vi "Sensor_Reference_Sensor_v1.1.vi"() -> ()   [LabVIEW 2012]
doc: "This example VI demonstrates setting up a scan list and taking a reading using the advanced VIs. For more information about the different types of VIs, see the descriptions below.\n\nEven though only two types of measurements are shown, all six types can be configured in the same way. Likewise, this VI does not show every available configurable option for voltage and resistance.\n\n====================\nSetting up and performing a scan\n====================\nThe HP34970A provides commands for setting up a scan in three ways that differ in their complexity and the amount of control offered:\n\n1. Advanced:\nEvery aspect of the measurement, scan, scan list, and read is put in a different command to allow the greatest flexibility. For example, using the advanced configure VIs, you can set up a scan list consisting of different measurement types on different channels. The \"HP34970A Advanced Scan Example.vi\" demonstrates usage of these VIs.\n\n2. Medium:\nThe instrument also offers a command that wraps up configuring individual channels and the scan list. This is represented in the driver by \"HP34970A Conf EZ.vi\". This driver specifically replaces use of the advanced configure measurement VIs and configure scan list VIs. For more information, refer to the context help for the Conf EZ VI.\n\n3. Easiest:\nThe entire configuration, scan, and read are wrapped up into one command to the instrument. This is provided in this driver as the \"EZ\" VIs, which are in the Data subpalette of the HP34970A's driver palette. The \"HP34970A EZ Scan Example.vi\" demonstrates the EZ VI's usage."
uses:
  <instrlib>/Agilent 34970/Agilent 34970.lvlib
  <vilib>/Analysis/NI_AALPro.lvlib
panel:
  in  "enable autozero":bool=TRUE
  out "real sampling time / ms":dbl[](array[numeric])
  out "size(s)":i32[](array[numeric])
  in  "Sample time set point / s":dbl=0.01
  out "max value":dbl
  out "Waveform Graph 2":T1(graph)
  out "read buffer":string
  in  "Scan Fields":T2={"Include Alarm Data F:(No)"=FALSE, "Include Channel # (F:No)"=FALSE, "Include Time (F:No)"=TRUE, "Include Units (F:No)"=FALSE}
  in  "number of readings":i32=3
  in  "Advanced Config":T3={"Aperture Value (.4)"=0.4, "Aperture (1:Minimum)"=1, "NPLC (1)"=2, "Bandwidth (3 Hz)"=0, "Input Impedance (F:Fixed)"=FALSE, "Integration Time (F:Aperture)"=TRUE} {"Aperture (1:Minimum)" items=["Manual", "Minimum", "Maximum"]; "NPLC (1)" items=[".02", ".2", "1", "2", "10", "20", "100", "200", "Minimum", "Maximum"]; "Bandwidth (3 Hz)" items=["3 Hz", "20 Hz", "200 Hz", "Minimum", "Maximum"]}
  out "measuring time / ms":u32
  out "measurement running":bool
  in  "current transfer ratio":dbl[unit]=1.0 caption="s"
  in  "Reading interval":u32=100
  in  "cancel measurement":bool
  out "standard deviation / %":dbl=nan format="%#_3g"
  out "mean / V":dbl format="%0.5f"
  out "standard deviation / V":dbl format="%0.5f"
  out "Waveform Graph":T1(graph)
  out "Readings":string[][](array[string])
  in  "Range (Volt.)":T4(ring)=enum."10 V"
  in  "Channel List (Volt.)":string="101"
  in  "VISA resource name":refnum<visa-resource-name>="USB0::0x0957::0x2007::MY49004365::INSTR"
  # "Voltage"
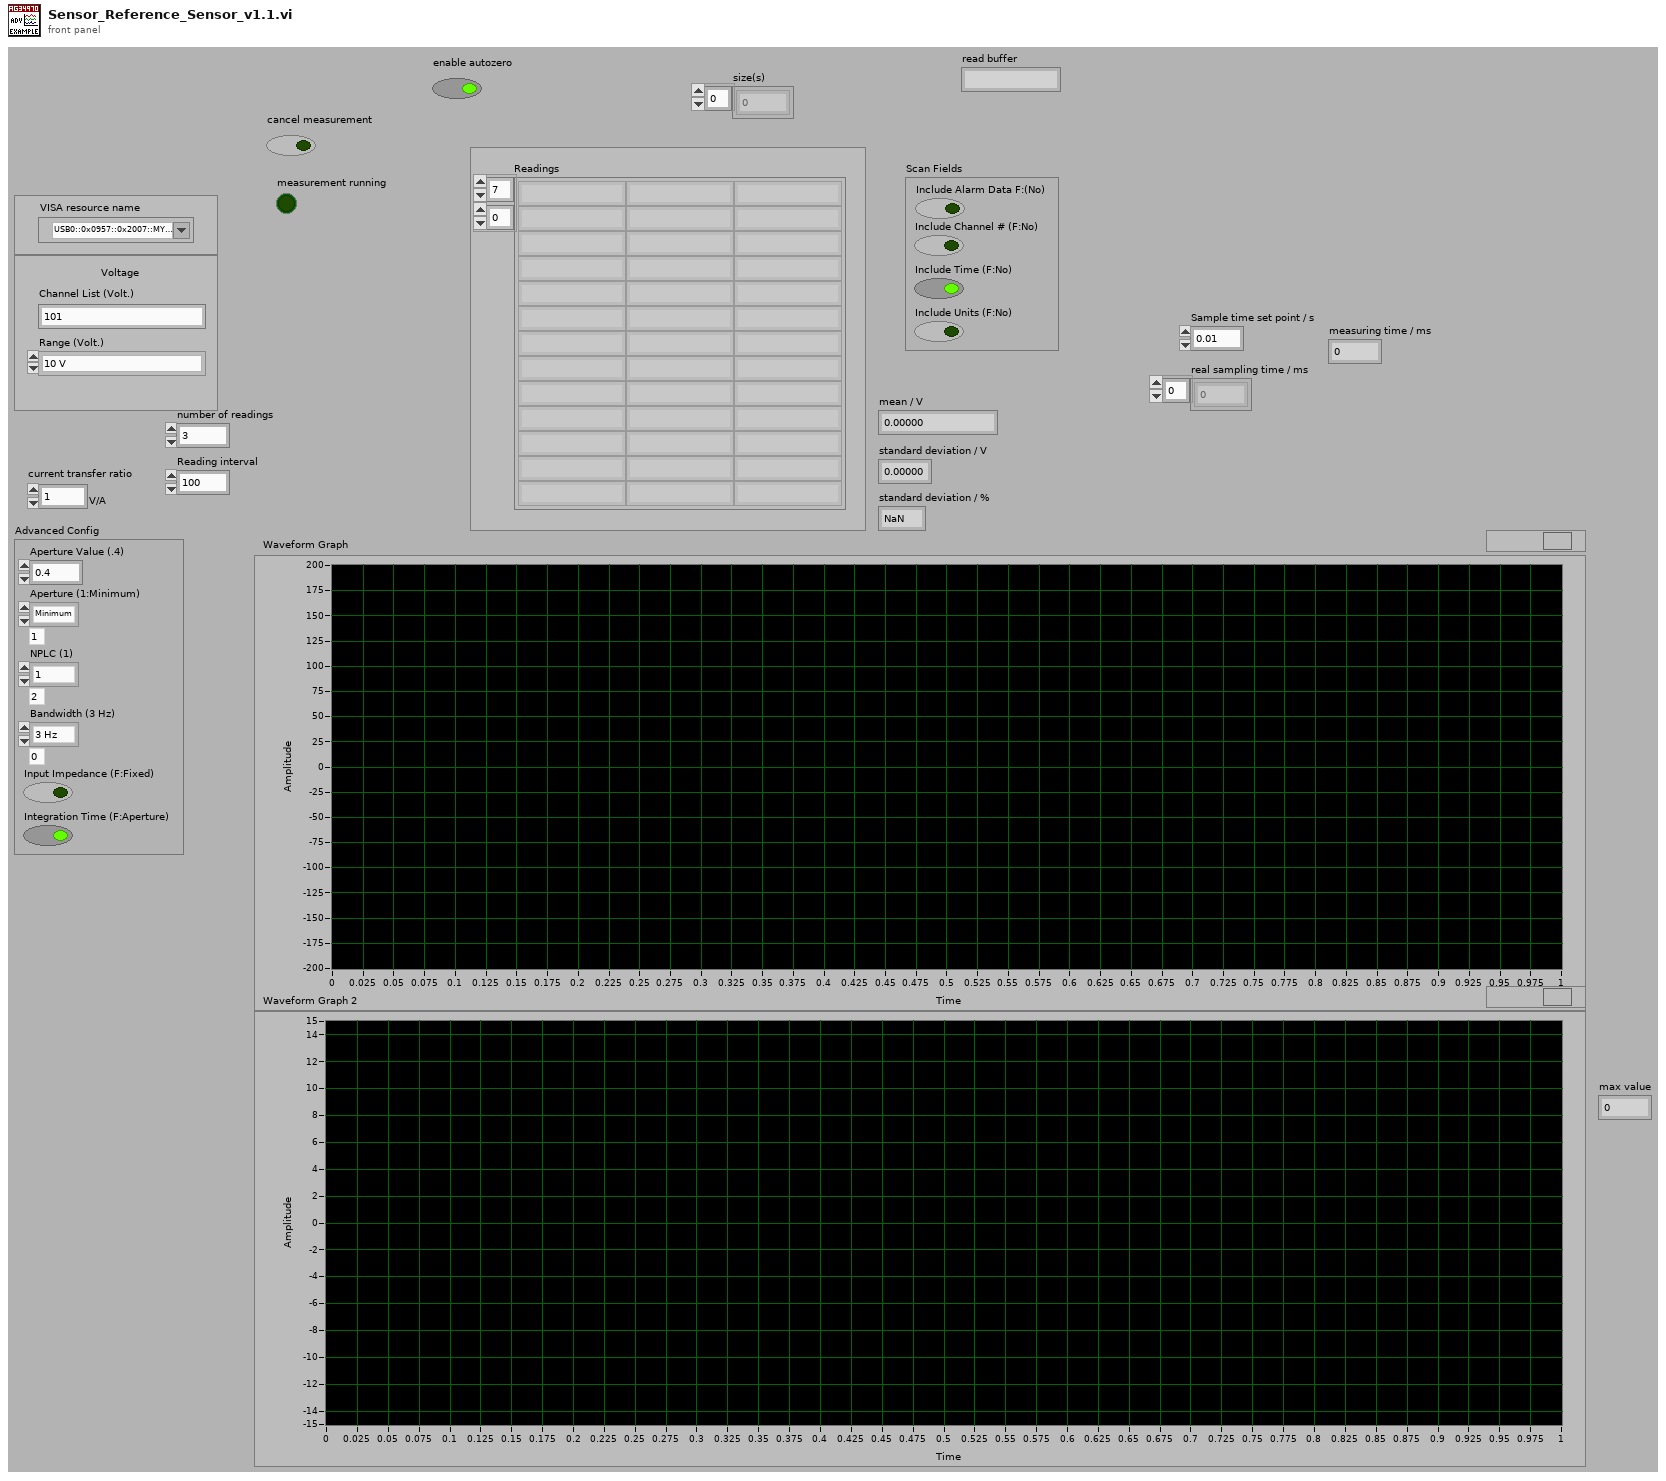
[diagram p1: front panel]
types:
  T1 = cluster{"Interval Value (0)":dbl, "Interval Value (0)":dbl, dbl[]}
  T2 = cluster{"Include Alarm Data F:(No)":bool, "Include Channel # (F:No)":bool, "Include Time (F:No)":bool, "Include Units (F:No)":bool}
  T3 = cluster{"Aperture Value (.4)":dbl, "Aperture (1:Minimum)":u16, "NPLC (1)":u16, "Bandwidth (3 Hz)":u16, "Input Impedance (F:Fixed)":bool, "Integration Time (F:Aperture)":bool}
  T4 = enum16{"100 mV", "1 V", "10 V", "100 V", "300 V", "Minimum", "Maximum"}
  T5 = enum16{"Manual", "Minimum", "Maximum", "Infinity"}
  T6 = enum16{"Remote Trigger", "Immediate Trigger", "Wait for Trigger", "Abort Scan"}
  T7 = enum16{"Bus", "Immediate", "External", "Alarm 1", "Alarm 2", "Alarm 3", "Alarm 4", "Timer"}
  T8 = cluster{"Timeout Value (10000)":u32, "Baud Rate (57600)":enum16{"1200", "2400", "4800", "9600", "19200", "38400", "57600", "115200"}, "Flow Control (1:XON/XOFF)":enum16{"None", "XON / XOFF", "RTS / CTS", "DTR / DSR"}}
  T9 = cluster{dbl, "Sample time set point / s":dbl, dbl[]}
  T10 = cluster{dbl, "Sample time set point / s":dbl, "dX/dt":dbl[]}
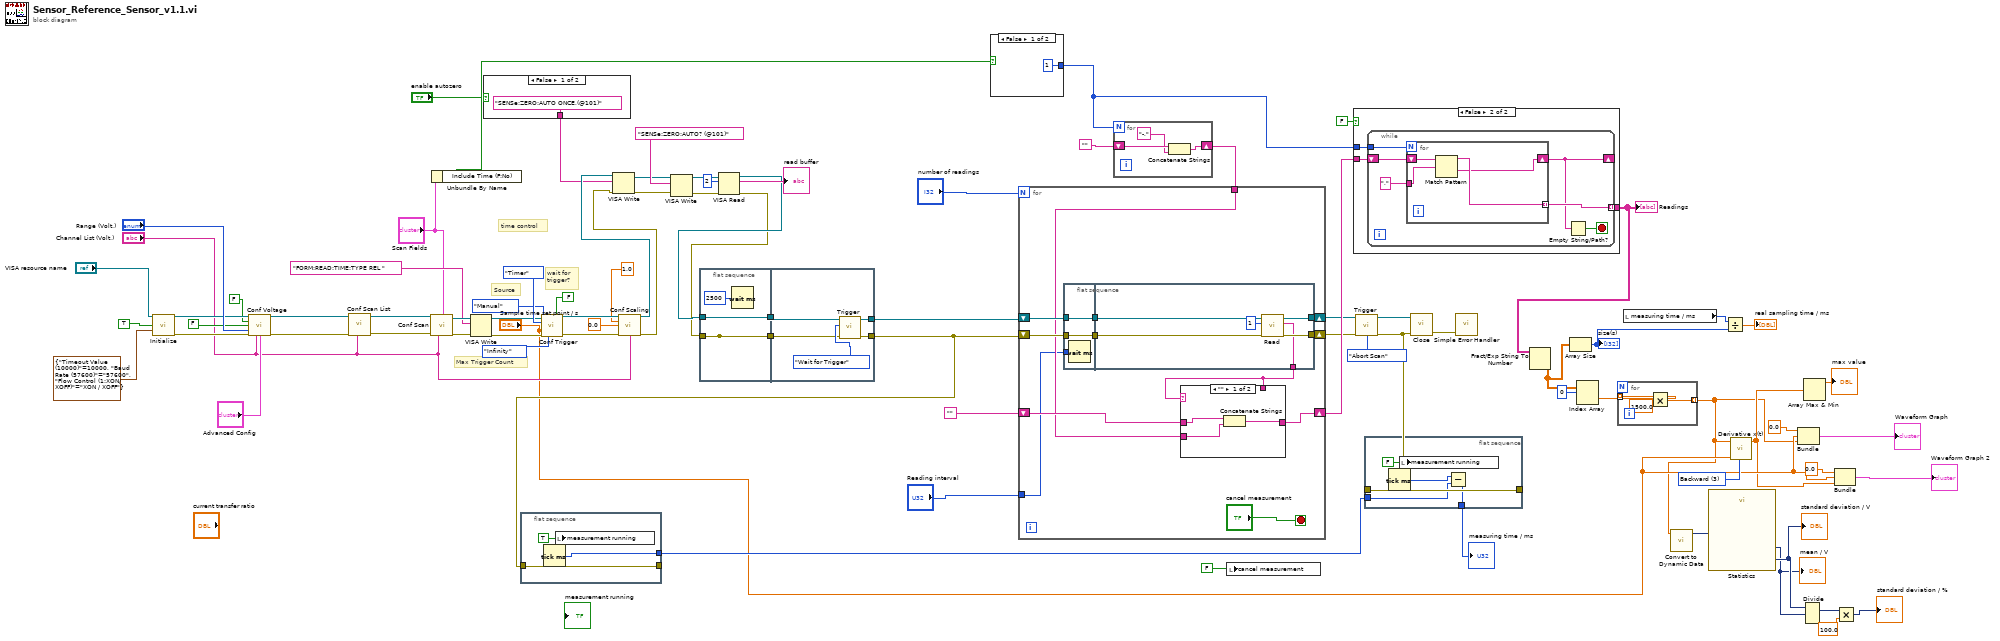
[diagram p0: block diagram]
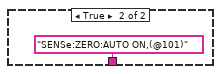
[diagram p2: hidden frame]
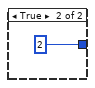
[diagram p3: hidden frame]
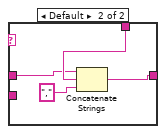
[diagram p4: hidden frame]
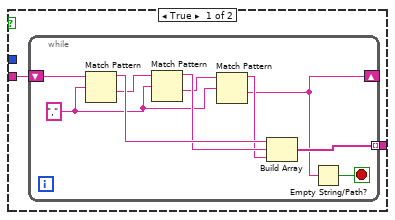
[diagram p5: hidden frame]
diagram:
  w11 = u16 3 items=["2nd Order Central", "4th Order Central", "Forward", "Backward"] ("method")
  # "Max Trigger Count"
  # "wait for \ntrigger?"
  # "time control"
  # "Source"
  n1 = call <instrlib>:"Initialize.vi"("VISA Resource Name"="VISA resource name", "Reset (T: Reset)"=TRUE, "Serial Port Configuration"=T8 {"Timeout Value (10000)"=10000, "Baud Rate (57600)"=enum."57600", "Flow Control (1:XON/XOFF)"=enum."XON / XOFF"}) -> ("VISA Resource Name Out"=w82:refnum<visa-resource-name>, "error out"=w69:errorcluster)  [unwired: 11 in]
  n2 = call <instrlib>:"Conf Voltage.vi"("VISA Resource Name"=w82, "AC/DC (F:DC)"=FALSE, "Autorange? (F:Off)"=FALSE, "Range (6:Max)"="Range (Volt.)", "error in (no error)"=w69, "Channel List (empty)"="Channel List (Volt.)", "Advanced Config"="Advanced Config") -> ("VISA Resource Name Out"=w71:refnum<visa-resource-name>, "error out"=w65:errorcluster)  [unwired: 6 in, 1 out]
  n3 = call <instrlib>:"Conf Scan List.vi"("Scan List (empty)"="Channel List (Volt.)", "error in (no error)"=w65, "VISA Resource Name"=w71) -> ("error out"=w64:errorcluster, "VISA Resource Name Out"=w67:refnum<visa-resource-name>)  [unwired: 6 in, 1 out]
  n4 = call <instrlib>:"Conf Scan.vi"("VISA Resource Name"=w67, "error in (no error)"=w64, "Channel List (empty)"="Channel List (Volt.)", "Scan Fields"="Scan Fields") -> ("VISA Resource Name Out"=w55:refnum<visa-resource-name>, "error out"=w54:errorcluster)  [unwired: 9 in, 1 out]
  n5 = Unbundle By Name("Scan Fields") -> ("Include Time (F:No)"=w37:bool)
  n6 = VISA Write(VISA resource name=w55, write buffer="FORM:READ:TIME:TYPE REL ", error in (no error)=w54) -> (VISA resource name out=w52:refnum<visa-resource-name>, error out=w53:errorcluster)  [unwired: 1 out]
  n7 = case shown="False" "enable autozero" {
    tunnel: ["SENSe:ZERO:AUTO ONCE,(@101)" ("write buffer") "SENSe:ZERO:AUTO ON,(@101)" ("write buffer")] -> w18
    frame False {
    }
    frame True {
    }
  }
  n8 = flat-sequence {
    tunnel: w35 -> [w89]
    tunnel: [w89] -> _
    tunnel: [w88] -> w57
    frame #0 {
      n9 = Tick Count (ms)() -> (millisecond timer value=w88:u32)
      n10 = local write "measurement running"(TRUE ("measurement running")) -> ()
    }
  }
  n11 = call <instrlib>:"Conf Trigger.vi"("VISA Resource Name"=w52, "Wait for Trigger? (F:No)"=FALSE, "Source (1:Immediate)"=T7."Timer", "Time-Scan Interval (1:Min)"=enum16{"Manual", "Minimum", "Maximum"}."Manual", "Interval Value (0)"="Sample time set point / s", "error in (no error)"=w53, "Max Trigger Count (3:Inf)"=T5."Infinity") -> ("VISA Resource Name Out"=w32:refnum<visa-resource-name>, "error out"=w31:errorcluster)  [unwired: 6 in, 1 out]
  n12 = call <instrlib>:"Conf Scaling.vi"("VISA Resource Name"=w32, "Gain (1)"=1.0, "Offset (0)"=0.0, "error in (no error)"=w31, "Channel List (empty)"="Channel List (Volt.)") -> ("VISA Resource Name Out"=w20:refnum<visa-resource-name>, "error out"=w19:errorcluster)  [unwired: 8 in, 1 out]
  n13 = VISA Write(VISA resource name=w20, write buffer=w18, error in (no error)=w19) -> (VISA resource name out=w22:refnum<visa-resource-name>, error out=w21:errorcluster)  [unwired: 1 out]
  n14 = VISA Write(VISA resource name=w22, write buffer="SENSe:ZERO:AUTO? (@101)", error in (no error)=w21) -> (VISA resource name out=w25:refnum<visa-resource-name>, error out=w24:errorcluster)  [unwired: 1 out]
  n15 = flat-sequence {
    tunnel: [w92] -> w17
    tunnel: w16 -> [w92]
    tunnel: [w91] -> _
    tunnel: [w91] -> w15
    tunnel: w14 -> [w91]
    tunnel: [w98] -> w36
    tunnel: [w97] -> w35
    tunnel: w17 -> [w95]
    tunnel: w15 -> [w94]
    frame #0 {
      n16 = Wait (ms)(milliseconds to wait=u32 2500) -> ()  [unwired: 1 out]
    }
    frame #1 {
      n17 = call <instrlib>:"Trigger.vi"("error in (no error)"=w94, "Command (0:Rem Trig)"=T6."Wait for Trigger", "VISA Resource Name"=w95) -> ("error out"=w97:errorcluster, "VISA Resource Name Out"=w98:refnum<visa-resource-name>)  [unwired: 7 in]
    }
  }
  n18 = VISA Read(VISA resource name=w25, byte count=u32 2, error in (no error)=w24) -> (VISA resource name out=w16:refnum<visa-resource-name>, read buffer=→"read buffer":string, error out=w14:errorcluster)  [unwired: 1 out]
  n19 = case shown="False" w37 {
    tunnel: [1 2] -> w41
    frame False {
    }
    frame True {
    }
  }
  n20 = for {
    N: w41 -> [_]
    shift-right: [w101] -> w39
    shift-left: "" -> [w103]
    n21 = Concatenate Strings(w103, "-," ("string")) -> (w101:string)
  }
  n22 = for {
    N: "number of readings" -> [_]
    shift-right: [w114] -> w81
    shift-left: "" -> [w113]
    tunnel: "Reading interval" -> [w104]
    shift-right: [w112] -> w46
    shift-left: w36 -> [w110]
    shift-right: [w115] -> w43
    shift-left: w35 -> [w109]
    tunnel: w39 -> [w107]
    stop <- "cancel measurement" stop-if-true
    n23 = flat-sequence {
      tunnel: w109 -> [w117]
      tunnel: w110 -> [w118]
      tunnel: [w118] -> w106
      tunnel: [w117] -> w105
      tunnel: w104 -> [w116]
      tunnel: [w124] -> w115
      tunnel: [w123] -> w112
      tunnel: [w120] -> w108
      tunnel: w106 -> [w122]
      tunnel: w105 -> [w121]
      frame #0 {
        n24 = Wait (ms)(milliseconds to wait=w116) -> ()  [unwired: 1 out]
      }
      frame #1 {
        n25 = call <instrlib>:"Read.vi"("error in (no error)"=w121, "# Channels (1)"=1, "VISA Resource Name"=w122) -> ("error out"=w124:errorcluster, "Readings"=w120:string, "VISA Resource Name Out"=w123:refnum<visa-resource-name>)  [unwired: 5 in, 1 out]
      }
    }
    n26 = case shown="\"\"" w108 {
      tunnel: [w127 w131] -> w114
      tunnel: w108 -> [_ w130]
      tunnel: w113 -> [w126 w129]
      tunnel: w107 -> [w125 _]
      frame "" {
        n27 = Concatenate Strings(w126, w125) -> (w127:string)
      }
      frame Default {
        n28 = Concatenate Strings(w129, w130, "," ("string")) -> (w131:string)
      }
    }
  }
  n29 = local write "cancel measurement"(FALSE ("Boolean")) -> ()
  n30 = case shown="False" FALSE {
    tunnel: w81 -> [w133 w146]
    tunnel: [w132 w145] -> w79
    tunnel: w41 -> [_ w144]
    frame True {
      n31 = while {
        tunnel: [w140] -> w132 mode=indexing
        shift-left: w133 -> [w143]
        shift-right: [w135] -> _
        stop <- w139 stop-if-true
        w134 = "," ("regular expression")
        n32 = Match Pattern(string=w143, regular expression=w134) -> (before substring=w142:string, after substring=w138:string)  [unwired: 1 in, 2 out]
        n33 = Match Pattern(string=w138, regular expression=w134) -> (before substring=w141:string, after substring=w137:string)  [unwired: 1 in, 2 out]
        n34 = Match Pattern(string=w137, regular expression=w134) -> (before substring=w136:string, after substring=w135:string)  [unwired: 1 in, 2 out]
        n35 = Build Array(w142, w141, w136) -> (w140:string[])
        n36 = Empty String/Path?(string/path=w135) -> (empty?=w139:bool)
      }
    }
    frame False {
      n37 = while {
        tunnel: [w151] -> w145 mode=indexing
        shift-left: w146 -> [w152]
        shift-right: [w148] -> _
        tunnel: w144 -> [w147]
        stop <- w150 stop-if-true
        n38 = for {
          N: w147 -> [_]
          tunnel: [w154] -> w151 mode=indexing
          tunnel: "," ("regular expression") -> [w155]
          shift-right: [w153] -> w148
          shift-left: w152 -> [w156]
          n39 = Match Pattern(string=w156, regular expression=w155) -> (before substring=w154:string, after substring=w153:string)  [unwired: 1 in, 2 out]
        }
        n40 = Empty String/Path?(string/path=w148) -> (empty?=w150:bool)
      }
    }
  }
  "Readings" <- w79
  n41 = call <instrlib>:"Trigger.vi"("error in (no error)"=w43, "Command (0:Rem Trig)"=T6."Abort Scan", "VISA Resource Name"=w46) -> ("error out"=w44:errorcluster, "VISA Resource Name Out"=w45:refnum<visa-resource-name>)  [unwired: 7 in]
  n42 = flat-sequence {
    tunnel: w44 -> [w160]
    tunnel: [w160] -> _
    tunnel: w57 -> [w158]
    tunnel: [w157] -> w56
    frame #0 {
      n43 = Tick Count (ms)() -> (millisecond timer value=w159:u32)
      n44 = local write "measurement running"(FALSE ("measurement running")) -> ()
      n45 = Subtract(x=w159, y=w158) -> (x-y=w157:u32)
    }
  }
  n46 = call <instrlib>:"Close.vi"("VISA Resource Name"=w45, "error in (no error)"=w44) -> ("error out"=w84:errorcluster)  [unwired: 13 in]
  n47 = call <vilib>:"Simple Error Handler.vi"("error in (no error)"=w84) -> ()  [unwired: 4 in, 5 out]
  n48 = Fract/Exp String To Number(string=w79) -> (number=w5:dbl[][])  [unwired: 3 in, 1 out]
  n49 = Array Size(array=w5) -> (size(s)=w3:i32[])
  "size(s)" <- w3
  n50 = Index Array(array=w5, index (col)=0 ("disabled index (col)")) -> (element=w6:dbl[])  [unwired: 1 in]
  n51 = for {
    tunnel: [w164] -> w7 mode=indexing
    tunnel: w6 -> [w163] mode=indexing
    n52 = Multiply(x=w163, y=1500.0) -> (x*y=w164:dbl)
  }
  n53 = local read "measuring time / ms"() -> (w4:u32)
  n54 = call "Convert to Dynamic Data"("Array"=w7) -> ("Dynamic Data Type"=w77:dynamicdata)  [unwired: 3 in]
  n55 = call "Statistics"("Signals"=w77) -> ("Standard Dev"=w76:dynamicdata, "Arithmetic Mean"=w75:dynamicdata)  [unwired: 24 in, 1 out]
  "standard deviation / V" <- w76
  "mean / V" <- w75
  n56 = Divide(x=w4, y=w3) -> (x/y=→"real sampling time / ms":dbl[])
  n57 = call <vilib>:"Derivative x(t).vi"("method"=w11, "dt"="Sample time set point / s", "X"=w7) -> ("dX/dt"=w9:dbl[])  [unwired: 7 in, 1 out]
  n58 = Bundle(0.0, "Sample time set point / s"="Sample time set point / s", w7) -> (→"Waveform Graph":T9)  [unwired: 1 in]
  n59 = Divide(1:w75, 2:w76) -> (0:w74:dynamicdata)  [unwired: 1 in, 1 out]
  n60 = Array Max & Min(array=w9) -> (max value=→"max value":dbl)  [unwired: 3 out]
  n61 = Bundle(0.0, "Sample time set point / s"="Sample time set point / s", "dX/dt"=w9) -> (→"Waveform Graph 2":T10)  [unwired: 1 in]
  n62 = Multiply(x=w74, y=100.0) -> (x*y=→"standard deviation / %":dynamicdata)
  "measuring time / ms" <- w56
